vi "DS345_BurstMode.get frequency.vi"(0 "i ref in":refnum<vi>, 5 "error in (no error)":errorcluster) -> (14 "i ref out":refnum<vi>, 15 "frequency [Hz}":dbl format="%.2f", 19 "error out":errorcluster)   [LabVIEW 2014, in "DS345_BurstMode.lvlib"]
doc: "Reads the frequency from the device"
uses:
  DS345_BurstMode.lvlib
  CSCore/CSSystem/CoreDefs/CoreDefs.error_type.ctl
  CSCore/CSSystem/CoreLib/CoreLib.lvlib
  CSCore/CSApplicationBaseClasses/AFGBase/AFGBase.lvlib
  CSCore/CSApplicationBaseClasses/DeviceBase/DeviceBase.lvlib
  CSCore/CSApplicationBaseClasses/AFGBase/AFGBase.directionType.ctl
  CSCore/CSApplicationBaseClasses/AFGBase/AFGBase.serviceType.ctl
  CSlibraries/UtilityLib/UtilityLib.valueStatus.ctl
  CSlibraries/UtilityLib/UtilityLib.lvlib
  CSCore/CSApplicationBaseClasses/DeviceBase/DeviceBase.deviceState.ctl
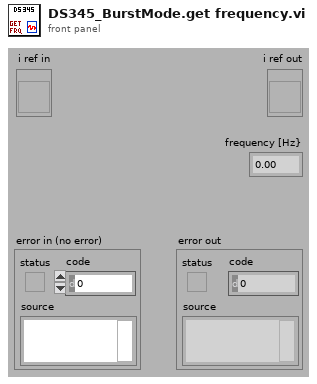
[diagram p1: front panel]
types:
  T1 = typedef "AFGBase.lvlib/AFGBase.serviceType.ctl" = enum16{"frequency", "amplitude", "phase", "DCOffset", "enableOutput", "trigger", "waveformType"}
  T2 = typedef "AFGBase.lvlib/AFGBase.directionType.ctl" = enum16{"unknown", "update actual value", "update nominal value", "update both"}
  T3 = typedef "UtilityLib.lvlib/UtilityLib.valueStatus.ctl" = enum16{"no info available", "stand by/off", "on", "warning", "alarm/malfunction", "not implemented", "user action required", "important information", "system default", "control default", "indicator default", "button default"}
  T4 = typedef "CoreDefs.error_type.ctl" = enum16{"no error", "can't load process", "can't unload process", "process does not exist", "can't install process", "can't remove process", "unknown function", "time out", "can't execute function", "duplicate queue name", "super not found", "caller queue invalid", "can't ping process", "unknown error", "VISA Error", "VISA timeout", "GPIB timeout", "GPIB error", "communication error", "data type mismatch", "can't read data from OPC server", "can't write data to OPC server", "OET error", "function not implemented", "process already exists", "invalid Shared Variable name", "error writing Shared Variable", "error reading Shared Variable", "invalid client name", "corrupt database", "unknown class", "call not authorized", "parameter out of range", "OET timeout: can't get data to modify", "invalid queue name", "requested operation incompatible with current state", "event undefined", "event disabled", "state undefined", "caller is not a friend", "EventBuilder: bad eventID", "EventBuilder: no DAQ devices", "a thread must not stop itself", "UNUSED ELEMENT4", "DiscArchiver: eventData incomplete", "DiscArchiver: eventData does not belong to run", "DiscArchiver: can't open file", "DiscArchiver: can't write to file", "DiscArchiver: available disc space low", "can't acquire semaphore", "error reading data from database", "notifier object is not existing", "can't register process", "can't unregister process", "illegal event type", "object disabled", "object already exists", "can't change state", "Instrument not found", "no connection to remote node", "invalid reference", "N/A", "UNUSED ELEMENT 1", "element not found", "illegal TCP/IP connection detected", "object does not exist", "invalid access ID", "unknown CS system", "invalid privilige", "unsupported data type", "unsupported server type", "IO server already exists", "Shared Variable already exists"}
  T5 = typedef "DeviceBase.lvlib/DeviceBase.deviceState.ctl" = i16
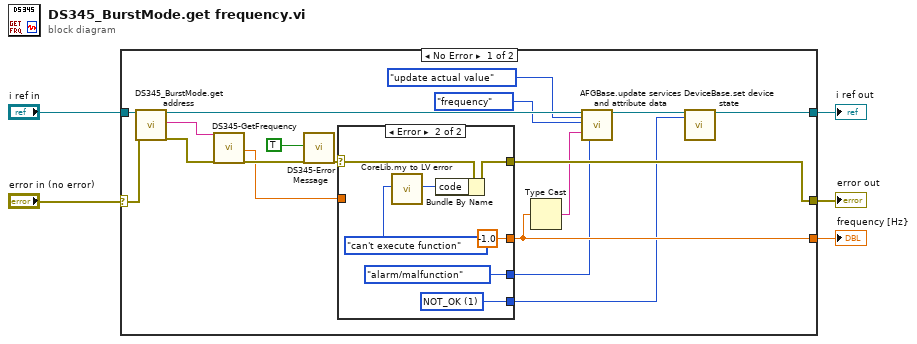
[diagram p0: block diagram]
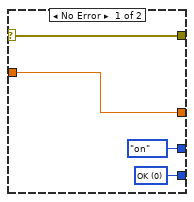
[diagram p2: hidden frame]
diagram:
  n1 = case shown="No Error" "error in (no error)" {
    selector: "error in (no error)" -> [w15 w35]
    tunnel: [w14 w35] -> w5
    tunnel: "i ref in" -> [w22 w36]
    tunnel: [w9 _] -> w3
    tunnel: [w12 w36] -> w2
    frame No Error {
      n2 = call "DS345_BurstMode.get address.vi"("i ref in"=w22, "error in (no error)"=w15) -> ("i ref out"=w16:refnum<vi>, "address"=w21:string, "error out"=w23:errorcluster)  [unwired: 15 in]
      n3 = call "DS345-GetFrequency.vi"("GPIB in"=w21, "error in (no error)"=w23) -> ("frequency [Hz]"=w17:dbl, "error out"=w20:errorcluster)  [unwired: 15 in, 1 out]
      n4 = call "DS345-Error Message.vi"("addMessageToSource"=TRUE ("add message to source"), "error in (no error)"=w20) -> ("error out"=w19:errorcluster)  [unwired: 14 in, 3 out]
      n5 = case shown="Error" w19 {
        selector: w19 -> [w27 w31]
        tunnel: [w27 w33] -> w14
        tunnel: [w26 -1.0 ("Frequency")] -> w9
        tunnel: w17 -> [w26 _]
        tunnel: [UtilityLib.valueStatus."on" ("quality") UtilityLib.valueStatus."alarm/malfunction" ("quality")] -> w7
        tunnel: [w24 w28] -> w6
        frame No Error {
          w24 = T5 0 items=["ERROR"=-1, "OK"=0, "NOT_OK"=1] ("deviceState")
        }
        frame Error {
          w28 = T5 1 items=["ERROR"=-1, "OK"=0, "NOT_OK"=1] ("deviceState")
          n6 = call "CoreLib.my to LV error.vi"("ErrorTypes"=CoreDefs.error_type."can't execute function") -> ("LV error code"=w32:i32)  [unwired: 17 in, 1 out]
          n7 = Bundle By Name(cluster=w31, "code"=w32) -> (w33:errorcluster)
        }
      }
      n8 = Type Cast(x=w9) -> (*(type *) &x=w8:string)  [unwired: 1 in]
      n9 = call "AFGBase.update services and attribute data.vi"("i ref in"=w16, "direction"=AFGBase.directionType."update actual value", "service"=AFGBase.serviceType."frequency", "value"=w8, "quality"=w7) -> ("i ref out"=w13:refnum<vi>)  [unwired: 12 in, 2 out]
      n10 = call "DeviceBase.set device state.vi"("i ref in"=w13, "deviceState"=w6) -> ("i ref out"=w12:refnum<vi>)  [unwired: 15 in, 2 out]
    }
    frame Error {
    }
  }
  "error out" <- w5
  "i ref out" <- w2
  "frequency [Hz}" <- w3
